vi "Micro-PL v10.4.0.vi"() -> ()   [LabVIEW 2010]
uses:
  drivers/Oxford ITC/ITCAPPS.LLB/ITCSetup.ctl
  drivers/Oxford ITC/ITCSUBS.LLB/ITCIO.ctl
  drivers/Oxford ITC/BUSGEN.LLB/OxfordAddress.ctl
  drivers/Oxford ITC/ITCSUBS.LLB/ITCVersion.ctl
  subvi/ESA-C/TypeDefs/ESA-C Live Controls.ctl
  subvi/ESA-C/TypeDefs/ESA-C Current Values.ctl
  subvi/ESA-C/TypeDefs/ESA-C Connection Settings.ctl
  subvi/ESA-C/TypeDefs/ESA-C Set Positions.ctl
  subvi/ITC503/TypeDefs/ITC503 Settings.ctl
  subvi/ITC503/TypeDefs/ITC503 Current Values.ctl
  subvi/iHR550/TypeDefs/iHR Current Values.ctl
  subvi/iHR550/TypeDefs/iHR Settings.ctl
  subvi/Mapping/TypeDefs/Mapping Spectra Params.ctl
  <vilib>/Utility/miscctls.llb/LVBoundsTypeDef.ctl
  <vilib>/Utility/miscctls.llb/LVPointTypeDef.ctl
  drivers/Horiba Spectrum One 3000V/Lib/CCD_command.llb/Comm Params.ctl
  subvi/Global Variables.vi
  <vilib>/Analysis/NI_AALBase.lvlib
panel:
  out "Spectrum Raw":dbl[][](array[numeric])
  out "Mapping State Storage":bool
  out "Mapping Reference":refnum<vi>
  out "Copy Drive Target":bool
  in  "CCD3500 Shutter":bool caption="Shutter:"
  out "ITC503 Temp Storage":dbl
  out "Runtime":u32
  out "ITC Gradient Time":i64
  out "Read ITC":bool
  out "Read CCD3500":bool
  out "Read iHR550":bool
  out "Read Drive":bool
  out "Spectrum Properties":cluster{"Position":T1, "Plot Area Size":T1}={"Position"={"Width"=36, "Height"=367}, "Plot Area Size"={"Width"=496, "Height"=264}}
  in  "Auto Folder":path caption="Ausgewählter Pfad"
  out "Int. Time Temp":dbl
  out "Wavelengths (nm)":dbl[](array[numeric])
  out "Measurement Running":bool
  out "ITC503s Running":bool
  out "Drive Running":bool
  out "CCD3500V Running":bool
  out "iHR550 Running":bool
  in  "Exit":bool
  out "iHR550 Status":bool
  out "Drive Status":bool
  out "CCD3500V Status":bool
  out "ITC503 Status":bool
  in  "CCD3500V Connection":T2={"Comm Interface"=1, "BUS"=0, "Address"=5, "Com Port"=0}
  out "Video Running":bool
  out "iHR550 RefNum":refnum<k7> caption="Mono RefNum out"
  out "ITC Setup":T3={"Description"="", "IO Info"={"Address"={"Com Port"=1, "ISOBUS Address"=1, "GPIB Address"=24, "Communication"=enum."ISOBUS"}, "Version"=enum."ITC503", "Ch 1 dec places"=1, "Ch 2 dec places"=1, "Ch 3 dec places"=1, "Ch1 Name"="", "Ch2 Name"="", "Ch3 Name"=""}}
  in  "Register":enum32{"Devices", "Acquisition / Mapping"}(tab)
  out "CCD3500 Temperature":dbl caption="Temp. (°C)" min=10.0 max=160.0 step=0.1 format="%.1f"
  in  "CCD3500V GPIB-Port":i32=5 caption="GPIB-Port" min=1 max=20 step=1 format="%#.0f"
  in  "CCD3500V Connect":bool
  out "CCD Timing":u32 caption="CCD"
  out "ITC Timing":u32 caption="ITC"
  out "Drive Timing":u32 caption="Drive"
  out "iHR550 Timing":u32 caption="iHR550"
  in  "iHR550 Force Init":bool=TRUE
  in  "iHR550 Connect":bool
  in  "iHR550 ID":string(combo)="iHR550" caption="Monochromator ID"
  out "ITC503 Current Values":T7 {"ITC503 Gradient" format="%.2f"; "ITC503 Setpoint" min=-273.0 max=300000.0 step=0.0001 format="%.1f"; "ITC503 I" format="%_1f"; "ITC503 P" format="%_1f"; "ITC503 Temperature" min=0.0 max=1645.0 step=1e-05 format="%.2f"; "ITC503 Heater" min=0.0 max=100.0 step=0.01 scale=0.0..100.0}
  in  "ITC503 Settings":T8={"ITC503 Set Setpoint"=0.0, "ITC503 Set Auto Heater"=TRUE, "ITC503 Set Auto PID"=TRUE, "P"=0.0, "I"=0.0, "D"=0.0} {"D" min=0.0 max=100.0 step=0.1 format="%.1f"; "I" min=0.0 max=100.0 step=0.1 format="%.1f"; "P" min=0.0 max=100.0 step=0.1 format="%.1f"; "ITC503 Set Setpoint" min=-273.0 max=300000.0 step=0.1 format="%.1f"}
  in  "ITC503 Configure":bool
  in  "ITC503 Connect":bool
  in  "ITC503 Selector":u16(ring) caption="Select Device" items=["ITC503s"]
  out "Drive Current Values":T9 {"Position"."Drive Z Position" min=-273.0 max=300000.0 step=0.0001 format="%.1f"; "Position"."Drive Y Position" min=-273.0 max=300000.0 step=0.0001 format="%.1f"; "Position"."Drive X Position" min=-273.0 max=300000.0 step=0.0001 format="%.1f"; "Voltages"."Drive Z Voltage" min=-273.0 max=300000.0 step=0.0001 format="%.1f"; "Voltages"."Drive Y Voltage" min=-273.0 max=300000.0 step=0.0001 format="%.1f"; "Voltages"."Drive X Voltage" min=-273.0 max=300000.0 step=0.0001 format="%.1f"}
  in  "Drive Connection":T10={"Objective GPIB-Port"=4, "Stage GPIB-Port"=4, "Drive Selector"=0, "Drive Velocity (V/s)"=5.0} {"Drive Velocity (V/s)" min=10.0 max=160.0 step=0.1 format="%.1f"; "Drive Selector" items=["Obj.", "Stage"]; "Stage GPIB-Port" min=1 max=20 step=1 format="%#.0f"; "Objective GPIB-Port" min=1 max=20 step=1 format="%#.0f"}
  in  "Drive Connect":bool
  in  "Spectrum Noise":i64 caption="Noise Level"
  in  "Wavelength Switch":bool
  out "Spectrum":cluster{dbl[], dbl[]}[](graph)
  in  "Spectrum Load":bool
  in  "Spectrum Save":bool
  in  "CCD3000 Current Rep.":string="0/0"
  in  "Spectrum Maximize":bool
  in  "Video Show":bool
  in  "Drive GoTo":bool caption="Objective Move Abs."
  in  "Drive New Positions":T11 {"Drive X Set" min=10.0 max=160.0 step=0.1 format="%.1f"; "Drive Z Set" min=10.0 max=160.0 step=0.1 format="%.1f"; "Drive Y Set" min=10.0 max=160.0 step=0.1 format="%.1f"}
  in  "Spectrum Autosave":bool caption="iHR550 Force Init"
  in  "CCD3500 Preview":bool
  in  "CCD3500 Acquire":bool
  in  "Spectra Settings":T12={"Integration Time"=1.0, "Repetitions"=1, "Mapping Spectra"=TRUE} caption="Mapping Spectra Settings" {"Repetitions" min=1 max=100 step=1; "Integration Time" min=0.1 max=6000.0 step=0.1 format="%.1f"}
  in  "Mapping Start":bool
  in  "iHR550 Configure":bool
  in  "iHR Settings":T13={"iHR550 Set Exit Mirror"=2, "iHR550 Set Side Exit"=0.0, "iHR550 Set Front Entrance"=0.0, "iHR550 Set Wavelength"=897.9988, "iHR550 Set Grating"=0, "iHR550 Set Grating Switch"=FALSE, "iHR550 Set Wavelength Switch"=FALSE, "iHR550 Set Mirror Switch"=FALSE, "iHR550 Set Slits Switch"=FALSE} {"iHR550 Set Grating" items=["1800"=1, "600"=2, "150"=3]; "iHR550 Set Wavelength" min=0.0 max=1500.0 step=1.0; "iHR550 Set Side Exit" min=0.0 max=2000.0 step=1.0; "iHR550 Set Exit Mirror" items=["Front"=2, "Side"=3]}
  out "iHR Current Values":T14={"iHR 550 Front Entrance"=0.0, "iHR550 Side Exit"=0.0, "iHR550 Wavelength"=897.9988, "iHR550 Exit Mirror"=2, "iHR550 Grating"="1", "Grating Index"=1} {"iHR550 Exit Mirror" items=["EntranceMirror", "ExitMirror", "Front", "Side"]}
  out "Drive Live Current Values":T9 {"Position"."Drive Z Position" min=-273.0 max=300000.0 step=0.0001 format="%.1f"; "Position"."Drive Y Position" min=-273.0 max=300000.0 step=0.0001 format="%.1f"; "Position"."Drive X Position" min=-273.0 max=300000.0 step=0.0001 format="%.1f"; "Voltages"."Drive Z Voltage" min=-273.0 max=300000.0 step=0.0001 format="%.1f"; "Voltages"."Drive Y Voltage" min=-273.0 max=300000.0 step=0.0001 format="%.1f"; "Voltages"."Drive X Voltage" min=-273.0 max=300000.0 step=0.0001 format="%.1f"}
  in  "Drive Live Controls":T15={"Snapshot"=FALSE, "Move Step"=1.0, "Move Home"=FALSE, "Move Down"=FALSE, "Move Up"=FALSE, "Move Left"=FALSE, "Move Right"=FALSE, "Move Out"=FALSE, "Move In"=FALSE} {"Move Step" min=0.0 max=30.0 step=0.1 format="%.1f"}
  # "Correlation Setup"
  # "Active"
  # "Active"
  # "ITC"
  # "iHR"
  # "Drive"
  # "CCD"
  # "Status"
  # "CCD"
  # "ITC"
  # "iHR"
  # "Drive"
  # "CCD"
  # "Timing"
  # "Monochromator"
  # "Cryostat"
  # "Drives"
  # "Drive Control"
  # "Spectrum"
  # "CCD"
  # "Mapping"
  # "Launch the Spectral Mapping VI and Raman Tool Set 2.0 in a new window."
  # "Monochromator"
  # "XY"
  # "Z"
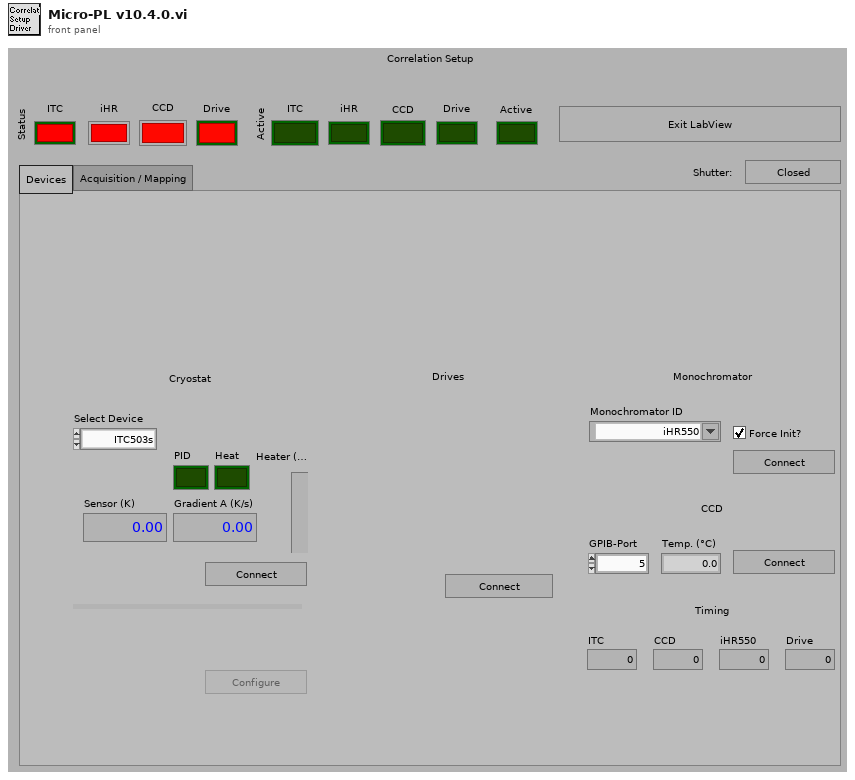
[diagram p1: front panel]
types:
  T1 = typedef "LVBoundsTypeDef.ctl" = cluster{"Width":u32, "Height":u32}
  T2 = cluster{"Comm Interface":u16, "BUS":i16, "Address":i16, "Com Port":i32}
  T3 = typedef "ITCSetup.ctl" = cluster{"Description":string, "IO Info":T4}
  T4 = typedef "ITCIO.ctl" = cluster{"Address":T5, "Version":T6, "Ch 1 dec places":i16, "Ch 2 dec places":i16, "Ch 3 dec places":i16, "Ch1 Name":string, "Ch2 Name":string, "Ch3 Name":string}
  T5 = typedef "OxfordAddress.ctl" = cluster{"Com Port":i32, "ISOBUS Address":i32, "GPIB Address":i16, "Communication":enum16{"RS232", "ISOBUS", "GPIB", "Gateway"}}
  T6 = typedef "ITCVersion.ctl" = enum16{"ITC502", "ITC503", "ITC601"}
  T7 = typedef "ITC503 Current Values.ctl" = cluster{"ITC503 Heater":dbl, "ITC503 Temperature":dbl, "ITC503 P":dbl, "ITC503 I":dbl, "ITC503 D":dbl, "ITC503 Setpoint":dbl, "ITC503 Gradient":dbl, "ITC503 Heater Auto":bool, "ITC503 PID Auto":bool}
  T8 = typedef "ITC503 Settings.ctl" = cluster{"ITC503 Set Setpoint":dbl, "ITC503 Set Auto Heater":bool, "ITC503 Set Auto PID":bool, "P":dbl, "I":dbl, "D":dbl}
  T9 = typedef "ESA-C Current Values.ctl" = cluster{"Voltages":cluster{"Drive X Voltage":dbl, "Drive Y Voltage":dbl, "Drive Z Voltage":dbl}, "Position":cluster{"Drive X Position":dbl, "Drive Y Position":dbl, "Drive Z Position":dbl}}
  T10 = typedef "ESA-C Connection Settings.ctl" = cluster{"Objective GPIB-Port":i32, "Stage GPIB-Port":i32, "Drive Selector":u16, "Drive Velocity (V/s)":dbl}
  T11 = typedef "ESA-C Set Positions.ctl" = cluster{"Drive X Set":dbl, "Drive Y Set":dbl, "Drive Z Set":dbl}
  T12 = typedef "Mapping Spectra Params.ctl" = cluster{"Integration Time":dbl, "Repetitions":u16, "Mapping Spectra":bool}
  T13 = typedef "iHR Settings.ctl" = cluster{"iHR550 Set Exit Mirror":u16, "iHR550 Set Side Exit":dbl, "iHR550 Set Front Entrance":dbl, "iHR550 Set Wavelength":dbl, "iHR550 Set Grating":u16, "iHR550 Set Grating Switch":bool, "iHR550 Set Wavelength Switch":bool, "iHR550 Set Mirror Switch":bool, "iHR550 Set Slits Switch":bool}
  T14 = typedef "iHR Current Values.ctl" = cluster{"iHR 550 Front Entrance":dbl, "iHR550 Side Exit":dbl, "iHR550 Wavelength":dbl, "iHR550 Exit Mirror":i32, "iHR550 Grating":string, "Grating Index":i32}
  T15 = typedef "ESA-C Live Controls.ctl" = cluster{"Snapshot":bool, "Move Step":dbl, "Move Home":bool, "Move Down":bool, "Move Up":bool, "Move Left":bool, "Move Right":bool, "Move Out":bool, "Move In":bool}
  T16 = typedef "LVPointTypeDef.ctl" = cluster{"Horizontal":i16, "Vertical":i16}
  T17 = enum8{"Enabled", "Disabled", "Disabled and Grayed Out"}
  T18 = typedef "Comm Params.ctl" = cluster{"Comm Interface":u16, "BUS":i16, "Address":i16, "Com Port":i32}
  T19 = enum16{"CCD Temperature Z345", "CCD Temperature Z308", "CCD Gain"}
  T20 = cluster{"CCD3000 Connection":T18, "Drive Connection Settings":T10, "ITC503 Current Values":T7, "Wavelengths (nm)":dbl[], "Drive Current Values":T9, "iHR Current Values":T14, "Spectra Settings":T12, "CCD3500 Temperature":dbl, "Simulate Drive 2":bool, "Simulate Spectra 2":bool}
  T21 = cluster{"Drive X Position":dbl, "Drive Y Position":dbl, "Drive Z Position":dbl}
  T22 = cluster{"Intensities":dbl[], "Wavelengths":dbl[]}[]
  T23 = typedef "LVPositionTypeDef.ctl" = cluster{"Left":i32, "Top":i32}
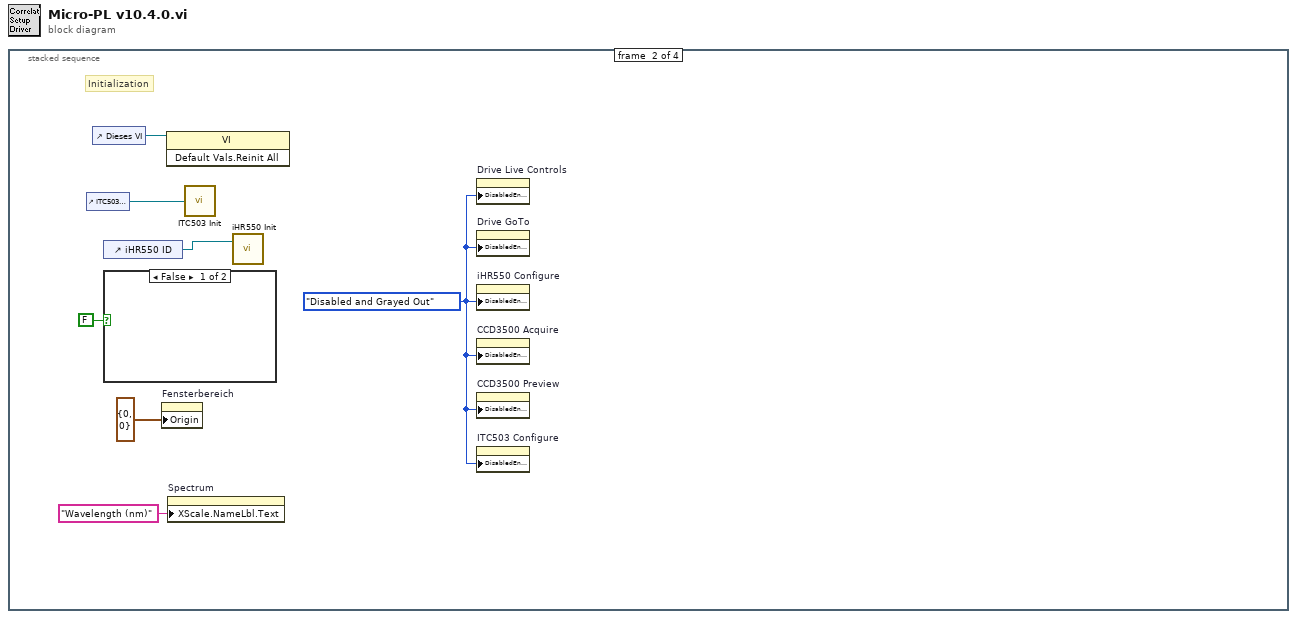
[diagram p0: block diagram]
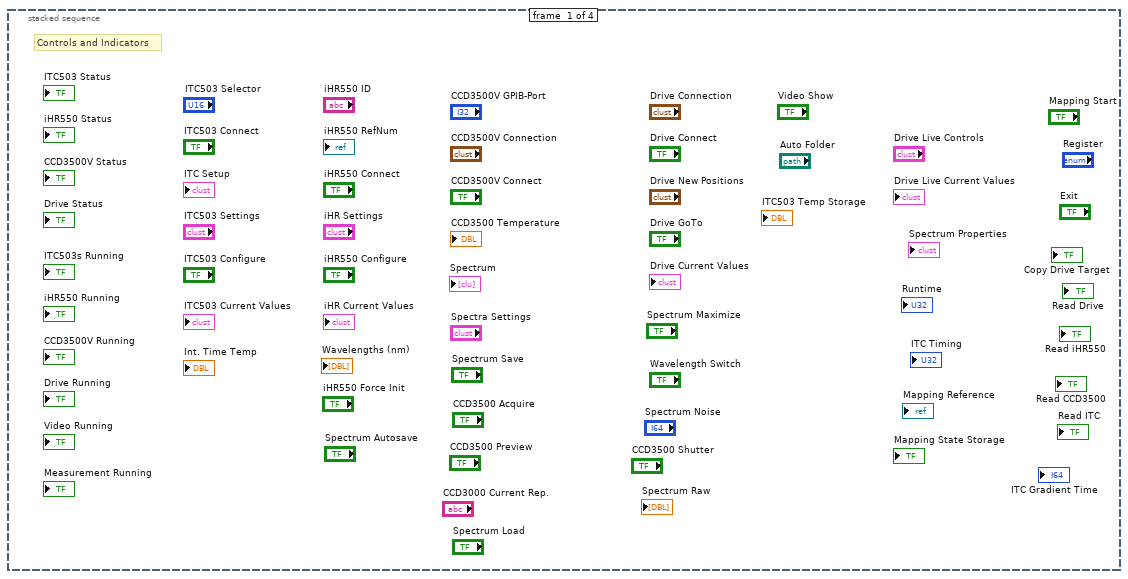
[diagram p2: hidden frame]
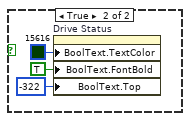
[diagram p3: hidden frame]
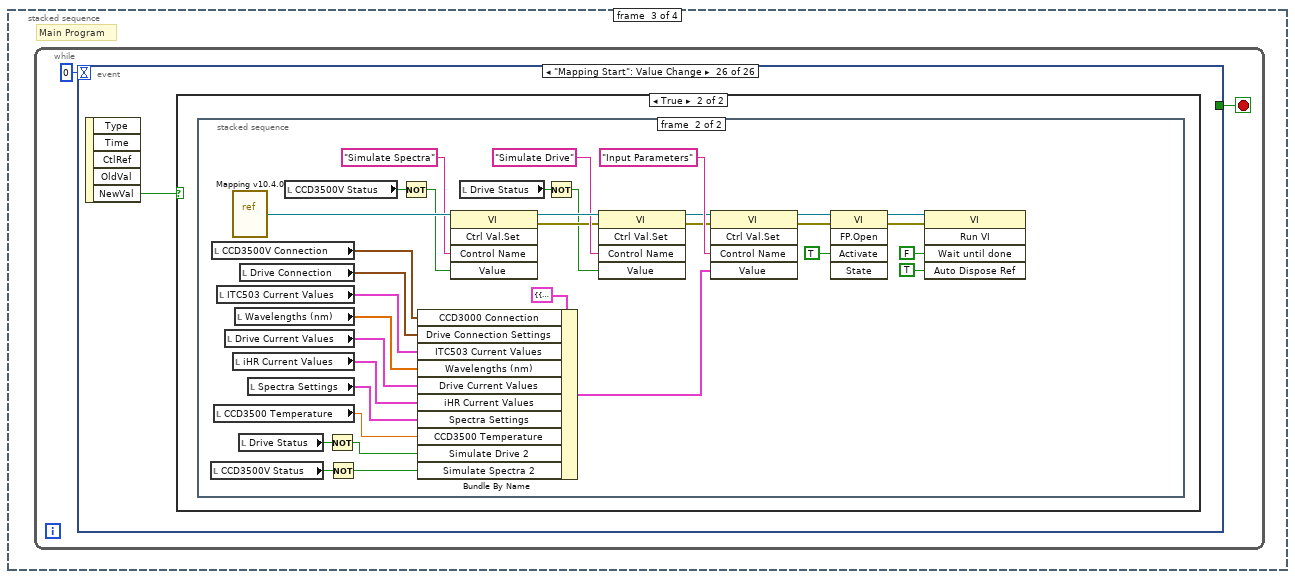
[diagram p4: hidden frame]
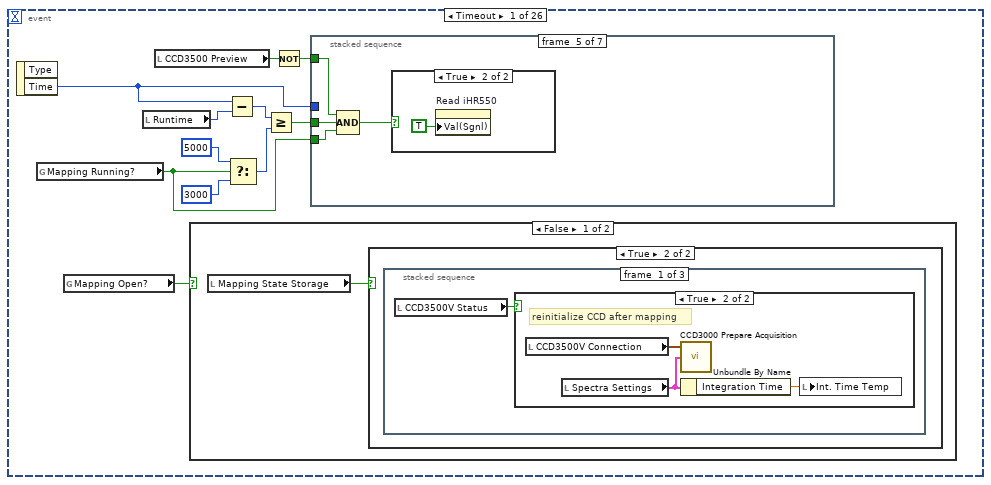
[diagram p5: hidden frame]
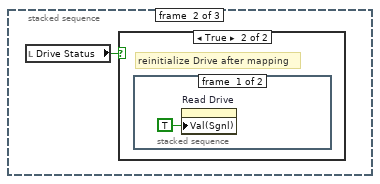
[diagram p8: hidden frame]
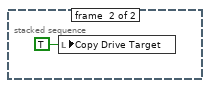
[diagram p10: hidden frame]
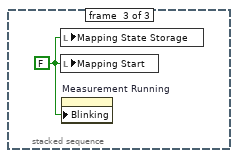
[diagram p11: hidden frame]
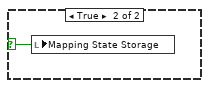
[diagram p12: hidden frame]
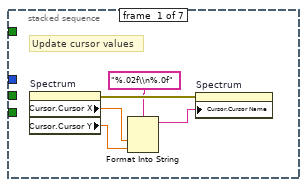
[diagram p13: hidden frame]
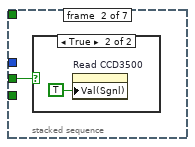
[diagram p14: hidden frame]
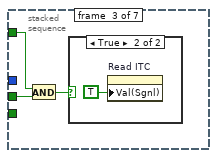
[diagram p16: hidden frame]
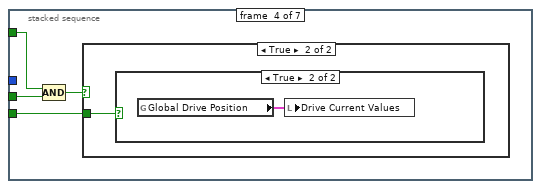
[diagram p18: hidden frame]
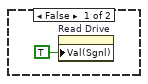
[diagram p20: hidden frame]
diagram:
  n1 = stacked-sequence {
    frame #0 {
      # "Controls and Indicators"
    }
    frame #1 {
      w2 = T17."Disabled and Grayed Out" ("Deaktiviert")
      # "Initialization"
      n2 = control-ref of="ITC503 Selector"() -> (w7:refnum<vi>)
      n3 = control-ref of="Dieses VI"() -> (w6:refnum<vi>)
      n4 = control-ref of="iHR550 ID"() -> (w5:refnum<vi>)
      n5 = case shown="False" FALSE {
        frame False {
        }
        frame True {
          n6 = property on="Drive Status" class="Bool (strict)"("BoolText.TextColor"=u32 15616, "BoolText.FontBold"=TRUE ("Boolescher Text.Schriftart:Fett"), "BoolText.Top"=-322 ("Boolescher Text.Position:Oben")) -> ()  [unwired: 2 in, 2 out]
        }
      }
      n7 = property on="Fensterbereich" class="Pane"("Origin"=T16 {"Horizontal"=0, "Vertical"=0}) -> ()  [unwired: 2 in, 2 out]
      n8 = invoke class="VI" method="Default Vals.Reinit All"(reference=w6) -> ()  [unwired: 2 in, 3 out]
      n9 = property on="Spectrum" class="XYGraph (strict)"("XScale.NameLbl.Text"="Wavelength (nm)" ("X Scale.Name Label.Text")) -> ()  [unwired: 2 in, 2 out]
      n10 = call "ITC503 Init.vi"("ITC Selector"=w7) -> ()  [unwired: 1 in]
      n11 = call "iHR550 Init.vi"("Mono ID"=w5) -> ()  [unwired: 2 in]
      n12 = property on="Drive Live Controls" class="Clust (strict)"("DisabledEnum"=w2) -> ()  [unwired: 2 in, 2 out]
      n13 = property on="Drive GoTo" class="Bool (strict)"("DisabledEnum"=w2) -> ()  [unwired: 2 in, 2 out]
      n14 = property on="iHR550 Configure" class="Bool (strict)"("DisabledEnum"=w2) -> ()  [unwired: 2 in, 2 out]
      n15 = property on="CCD3500 Acquire" class="Bool (strict)"("DisabledEnum"=w2) -> ()  [unwired: 2 in, 2 out]
      n16 = property on="CCD3500 Preview" class="Bool (strict)"("DisabledEnum"=w2) -> ()  [unwired: 2 in, 2 out]
      n17 = property on="ITC503 Configure" class="Bool (strict)"("DisabledEnum"=w2) -> ()  [unwired: 2 in, 2 out]
    }
    frame #2 {
      # "Main Program"
      n18 = while "Main-Program" {
        stop <- w12 stop-if-true
        n19 = event shown="[25] \"Mapping Start\": Value Change" {
          selector: _ -> [_ _ _ _ _ _ _ _ _ _ _ _ _ _ _ _ _ _ _ _ _ _ _ _ _ _]
          dyn-events: _ -> [_ _ _ _ _ _ _ _ _ _ _ _ _ _ _ _ _ _ _ _ _ _ _ _ _ _]
          timeout: 0 -> [_ _ _ _ _ _ _ _ _ _ _ _ _ _ _ _ _ _ _ _ _ _ _ _ _ _]
          tunnel: [_ w62 _ _ _ _ _ _ _ _ _ _ _ _ _ _ _ _ _ _ _ _ _ _ _ _] -> w12
          event Timeout {
            n20 = event-data() -> ("Time"=w19:u32)  [unwired: 1 in, 1 out]
            n21 = global read "Global Variables.vi" "Mapping Running?"() -> (w14:bool)
            n22 = global read "Global Variables.vi" "Mapping Open?"() -> (w13:bool)
            n23 = local read "Runtime"() -> (w18:u32)
            n24 = local read "CCD3500 Preview"() -> (w21:bool)
            n25 = case shown="False" w13 {
              selector: w13 -> [_ w33]
              frame False {
                n26 = local read "Mapping State Storage"() -> (w24:bool)
                n27 = case shown="True" w24 {
                  frame False {
                  }
                  frame True {
                    n28 = stacked-sequence {
                      frame #0 {
                        n29 = local read "CCD3500V Status"() -> (w25:bool)
                        n30 = case shown="True" w25 {
                          frame False {
                          }
                          frame True {
                            # "reinitialize CCD after mapping"
                            n31 = local read "CCD3500V Connection"() -> (w26:T2)
                            n32 = local read "Spectra Settings"() -> (w28:T12)
                            n33 = call "CCD3000 Prepare Acquisition.vi"("Mapping Spectra Settings"=w28, "Comm Params"=w26) -> ()  [unwired: 4 in]
                            n34 = Unbundle By Name(w28) -> ("Integration Time"=w27:dbl)
                            n35 = local write "Int. Time Temp"(w27) -> ()
                          }
                        }
                      }
                      frame #1 {
                        n36 = local read "Drive Status"() -> (w29:bool)
                        n37 = case shown="True" w29 {
                          frame False {
                          }
                          frame True {
                            # "reinitialize Drive after mapping"
                            n38 = stacked-sequence {
                              frame #0 {
                                n39 = property on="Read Drive" class="Bool (strict)"("Val(Sgnl)"=TRUE ("Value (Signaling)")) -> ()  [unwired: 2 in, 2 out]
                              }
                              frame #1 {
                                n40 = local write "Copy Drive Target"(TRUE ("Copy Drive Target")) -> ()
                              }
                            }
                          }
                        }
                      }
                      frame #2 {
                        w32 = FALSE ("Mapping Start")
                        n41 = local write "Mapping State Storage"(w32) -> ()
                        n42 = local write "Mapping Start"(w32) -> ()
                        n43 = property on="Measurement Running" class="Bool (strict)"("Blinking"=w32) -> ()  [unwired: 2 in, 2 out]
                      }
                    }
                  }
                }
              }
              frame True {
                n44 = local write "Mapping State Storage"(w33) -> ()
              }
            }
            n45 = Subtract(x=w19, y=w18) -> (x-y=w22:u32)
            n46 = Select(t=u32 5000 ("y"), s=w14, f=u32 3000 ("y")) -> (s? t:f=w15:u32)
            n47 = Greater Or Equal?(x=w22, y=w15) -> (x >= y?=w23:bool)
            n48 = Not(x=w21) -> (.not. x?=w20:bool)
            n49 = stacked-sequence {
              tunnel: w23 -> [_ w39 w43 w48 w55 _ w59]
              tunnel: w19 -> [_ _ _ _ _ _ w60]
              tunnel: w20 -> [_ _ w42 w47 w54 w57 _]
              tunnel: w14 -> [_ _ _ w45 w52 _ _]
              frame #0 {
                # "Update cursor values"
                n50 = property on="Spectrum" class="XYGraph (strict)"() -> (error out=w38:errorcluster, "Cursor.Cursor X"=w37:dbl, "Cursor.Cursor Y"=w36:dbl)  [unwired: 2 in, 1 out]
                n51 = Format Into String(format string="%.02f\\n%.0f", w37, w36) -> (resulting string=w34:string)  [unwired: 2 in, 1 out]
                n52 = property on="Spectrum" class="XYGraph (strict)"(error in=w38, "Cursor.Cursor Name"=w34) -> ()  [unwired: 1 in, 2 out]
              }
              frame #1 {
                n53 = case shown="True" w39 {
                  frame False {
                  }
                  frame True {
                    n54 = property on="Read CCD3500" class="Bool (strict)"("Val(Sgnl)"=TRUE ("Value (Signaling)")) -> ()  [unwired: 2 in, 2 out]
                  }
                }
              }
              frame #2 {
                n55 = And(x=w42, y=w43) -> (x .and. y?=w41:bool)
                n56 = case shown="True" w41 {
                  frame False {
                  }
                  frame True {
                    n57 = property on="Read ITC" class="Bool (strict)"("Val(Sgnl)"=TRUE ("Value (Signaling)")) -> ()  [unwired: 2 in, 2 out]
                  }
                }
              }
              frame #3 {
                n58 = Compound Arithmetic op=AND(w47, w48) -> (w46:bool)
                n59 = case shown="True" w46 {
                  tunnel: w45 -> [_ w49]
                  frame False {
                  }
                  frame True {
                    n60 = case shown="True" w49 {
                      frame False {
                        n61 = property on="Read Drive" class="Bool (strict)"("Val(Sgnl)"=TRUE ("Value (Signaling)")) -> ()  [unwired: 2 in, 2 out]
                      }
                      frame True {
                        n62 = global read "Global Variables.vi" "Global Drive Position"() -> (w51:T9)
                        n63 = local write "Drive Current Values"(w51) -> ()
                      }
                    }
                  }
                }
              }
              frame #4 {
                n64 = Compound Arithmetic op=AND(w54, w55, w52) -> (w53:bool)
                n65 = case shown="True" w53 {
                  frame False {
                  }
                  frame True {
                    n66 = property on="Read iHR550" class="Bool (strict)"("Val(Sgnl)"=TRUE ("Value (Signaling)")) -> ()  [unwired: 2 in, 2 out]
                  }
                }
              }
              frame #5 {
                n67 = case shown="False" w57 {
                  frame False {
                    n68 = property on="CCD3500 Acquire" class="Bool (strict)"("Val(Sgnl)"=TRUE ("Wert (signalisierend)")) -> ()  [unwired: 2 in, 2 out]
                  }
                  frame True {
                  }
                }
              }
              frame #6 {
                # "Set runtime counter"
                n69 = case shown="True" w59 {
                  tunnel: w60 -> [_ w61]
                  frame False {
                  }
                  frame True {
                    n70 = local write "Runtime"(w61) -> ()
                  }
                }
              }
            }
          }
          event "Exit": Value Change {
            n71 = event-data() -> ("NewVal"=w62:bool)  [unwired: 1 in, 4 out]
          }
          event "ITC503 Connect": Value Change {
            n72 = event-data() -> ("NewVal"=w63:bool)  [unwired: 1 in, 4 out]
            n73 = stacked-sequence {
              tunnel: w63 -> [_ w65 _]
              frame #0 {
                n74 = property on="ITC503s Running" class="Bool (strict)"("Blinking"=TRUE ("Blinkend")) -> ()  [unwired: 2 in, 2 out]
              }
              frame #1 {
                n75 = case shown="True" w65 {
                  selector: w65 -> [w70 _]
                  tunnel: [w70 w77] -> w67
                  frame False {
                    # "disconnect"
                    n76 = control-ref of="ITC503s Running"() -> (w71:refnum<vi>)
                    n77 = property class="Bool (strict)"(reference=w71, "Blinking"=w70, "Value"=w70) -> ()  [unwired: 1 in, 2 out]
                  }
                  frame True {
                    # "connect"
                    n78 = local read "ITC503 Selector"() -> (w78:u16)
                    n79 = call "ITC503 Connect.vi"("ITC Selector"=w78) -> ("ITC Setup"=w76:T3, "Connected"=w77:bool)
                    n80 = local write "ITC Setup"(w76) -> ()
                    n81 = call "ITC503 Get Values.vi"("ITC Setup"=w76) -> ("ITC503 Current Values"=w75:T7)  [unwired: 1 in, 1 out]
                    n82 = Unbundle By Name(w75) -> ("ITC503 Setpoint"=w72:dbl)
                    n83 = Bundle By Name(cluster=T8 {"ITC503 Set Setpoint"=0.0, "ITC503 Set Auto Heater"=TRUE, "ITC503 Set Auto PID"=TRUE, "P"=0.0, "I"=0.0, "D"=0.0} ("ITC503 Settings"), "ITC503 Set Setpoint"=w72) -> (w73:T8)
                    n84 = local write "ITC503 Settings"(w73) -> ()
                  }
                }
                n85 = case shown="False" w67 {
                  tunnel: [T17."Disabled and Grayed Out" ("Deaktiviert") T17."Enabled" ("Deaktiviert")] -> w66
                  frame False {
                  }
                  frame True {
                  }
                }
                n86 = local write "ITC503 Status"(w67) -> ()
                n87 = local write "ITC503 Connect"(w67) -> ()
                n88 = property on="ITC503 Configure" class="Bool (strict)"("DisabledEnum"=w66) -> ()  [unwired: 2 in, 2 out]
              }
              frame #2 {
                n89 = property on="ITC503s Running" class="Bool (strict)"("Blinking"=FALSE ("Blinkend")) -> ()  [unwired: 2 in, 2 out]
                n90 = property on="Read ITC" class="Bool (strict)"("Val(Sgnl)"=TRUE ("Wert (signalisierend)")) -> ()  [unwired: 2 in, 2 out]
              }
            }
          }
          event "Read ITC": Value Change {
            n91 = event-data() -> ("Time"=w82:u32, "NewVal"=w86:bool)  [unwired: 1 in, 3 out]
            n92 = local read "ITC503 Status"() -> (w85:bool)
            n93 = control-ref of="ITC503s Running"() -> (w83:refnum<vi>)
            n94 = And(x=w85, y=w86) -> (x .and. y?=w84:bool)
            n95 = case shown="True" w84 {
              tunnel: w83 -> [w88 w92]
              tunnel: w82 -> [_ w91]
              tunnel: [u32 0 w90] -> w81
              frame False {
                n96 = property class="Bool (strict)"(reference=w88, "BoolText.Text"="" ("Boolescher Text.Text")) -> ()  [unwired: 1 in, 2 out]
              }
              frame True {
                n97 = stacked-sequence {
                  seq-local: [_ w98 _ _] -> [_ _ w114 _]
                  seq-local: [w93 _ _ _] -> [_ _ _ w120]
                  tunnel: w92 -> [_ _ w107 _]
                  tunnel: w91 -> [_ w99 _ _]
                  tunnel: [_ _ _ w121] -> w90
                  frame #0 {
                    n98 = Tick Count (ms)() -> (millisecond timer value=w93:u32)
                  }
                  frame #1 {
                    n99 = local read "ITC Setup"() -> (w105:T3)
                    n100 = local read "ITC Gradient Time"() -> (w103:i64)
                    n101 = call "ITC503 Get Values.vi"("ITC Setup"=w105) -> ("ITC503 Current Values"=w98:T7)  [unwired: 1 in, 1 out]
                    n102 = local read "ITC503 Temp Storage"() -> (w97:dbl)
                    n103 = Unbundle By Name(w98) -> ("ITC503 Temperature"=w95:dbl)
                    n104 = Subtract(x=w99, y=w103) -> (x-y=w102:i64)
                    n105 = Divide(x=w102, y=i64 1000) -> (x/y=w100:dbl)
                    n106 = Subtract(x=w95, y=w97) -> (x-y=w96:dbl)
                    n107 = Divide(x=w96, y=w100) -> (x/y=w104:dbl)
                    n108 = Bundle By Name(cluster=w98, "ITC503 Gradient"=w104) -> (w94:T7)
                    n109 = local write "ITC503 Current Values"(w94) -> ()
                    n110 = global write "Global Variables.vi" "Global ITC Values"(w94) -> ()
                  }
                  frame #2 {
                    n111 = Unbundle By Name(w114) -> ("ITC503 Temperature"=w106:dbl, "ITC503 Setpoint"=w115:dbl)
                    n112 = Subtract(x=w106, y=w115) -> (x-y=w116:dbl)
                    n113 = Number To Fractional String(number=w106, precision (6)=i16 2 ("Genauigkeit (6)")) -> (F-format string=w110:string)  [unwired: 2 in]
                    n114 = Absolute Value(x=w116) -> (abs(x)=w117:dbl)
                    n115 = String Subset(string=w110, length (rest)=5 ("Länge (Rest)")) -> (substring=w108:string)  [unwired: 1 in]
                    n116 = Greater?(x=w117, y=2.0) -> (0:w113:bool)
                    n117 = Not(x=w113) -> (.not. x?=w112:bool)
                    n118 = property class="Bool (strict)"(reference=w107, "Blinking"=w113, "Value"=w112, "BoolText.Text"=w108) -> ()  [unwired: 1 in, 2 out]
                    n119 = local write "ITC503 Temp Storage"(w106) -> ()
                  }
                  frame #3 {
                    n120 = Tick Count (ms)() -> (millisecond timer value=w119:u32)
                    n121 = local write "ITC Gradient Time"(w119) -> ()
                    n122 = Subtract(x=w119, y=w120) -> (x-y=w121:u32)
                  }
                }
              }
            }
            n123 = local write "ITC Timing"(w81) -> ()
          }
          event "iHR550 Connect": Value Change {
            n124 = event-data() -> ("NewVal"=w122:bool)  [unwired: 1 in, 4 out]
            n125 = stacked-sequence {
              tunnel: w122 -> [_ w125 _]
              frame #0 {
                n126 = property on="iHR550 Running" class="Bool (strict)"("Blinking"=TRUE ("Blinkend")) -> ()  [unwired: 2 in, 2 out]
              }
              frame #1 {
                n127 = case shown="True" w125 {
                  selector: w125 -> [w129 _]
                  tunnel: [w129 w142] -> w124
                  frame False {
                    # "disconnect"
                  }
                  frame True {
                    # "connect"
                    n128 = local read "iHR550 Force Init"() -> (w140:bool)
                    n129 = control-ref of="iHR550 Set Grating"() -> (w141:refnum<vi>)
                    n130 = local read "iHR550 ID"() -> (w143:string)
                    n131 = call "iHR550 Connect.vi"("Force\nInitialization"=w140, "Grating Selector"=w141, "Mono ID"=w143) -> ("Initialized"=w142:bool, "iHR550 RefNum"=w139:refnum<k7>)  [unwired: 2 in, 4 out]
                    n132 = local write "iHR550 RefNum"(w139) -> ()
                    n133 = call "iHR550 Read Values.vi"("JYMONOLib.IJYMonoReqd"=w139) -> ("iHR Current Values"=w131:T14)  [unwired: 1 in]
                    n134 = local write "iHR Current Values"(w131) -> ()
                    n135 = Unbundle By Name(w131) -> ("iHR 550 Front Entrance"=w137:dbl, "iHR550 Side Exit"=w136:dbl, "iHR550 Wavelength"=w135:dbl, "iHR550 Exit Mirror"=w134:i32, "Grating Index"=w132:i32)
                    n136 = call "iHR550 Convert Axis.vi"("iHR Current Values"=w131) -> ("Wavelengths (nm)"=w130:dbl[])
                    n137 = local write "Wavelengths (nm)"(w130) -> ()
                    n138 = Bundle By Name(cluster=T13 {"iHR550 Set Exit Mirror"=0, "iHR550 Set Side Exit"=0.0, "iHR550 Set Front Entrance"=0.0, "iHR550 Set Wavelength"=0.0, "iHR550 Set Grating"=0, "iHR550 Set Grating Switch"=FALSE, "iHR550 Set Wavelength Switch"=FALSE, "iHR550 Set Mirror Switch"=FALSE, "iHR550 Set Slits Switch"=FALSE} ("iHR Settings"), "iHR550 Set Front Entrance"=w137, "iHR550 Set Side Exit"=w136, "iHR550 Set Wavelength"=w135, "iHR550 Set Exit Mirror"=w134, "iHR550 Set Grating"=w132) -> (w133:T13)
                    n139 = local write "iHR Settings"(w133) -> ()
                  }
                }
                n140 = local write "iHR550 Status"(w124) -> ()
                n141 = local write "iHR550 Connect"(w124) -> ()
                n142 = case shown="False" w124 {
                  tunnel: [T17."Disabled and Grayed Out" ("Deaktiviert") T17."Enabled" ("Deaktiviert")] -> w126
                  frame False {
                  }
                  frame True {
                  }
                }
                n143 = property on="iHR550 Configure" class="Bool (strict)"("DisabledEnum"=w126) -> ()  [unwired: 2 in, 2 out]
              }
              frame #2 {
                n144 = local write "iHR550 Force Init"(FALSE ("iHR550 Force Init")) -> ()
                n145 = property on="iHR550 Running" class="Bool (strict)"("Blinking"=FALSE ("Blinkend")) -> ()  [unwired: 2 in, 2 out]
                n146 = property on="Read iHR550" class="Bool (strict)"("Val(Sgnl)"=TRUE ("Wert (signalisierend)")) -> ()  [unwired: 2 in, 2 out]
              }
            }
          }
          event "Read iHR550": Value Change {
            n147 = event-data() -> ("NewVal"=w150:bool)  [unwired: 1 in, 4 out]
            n148 = local read "iHR550 Status"() -> (w149:bool)
            n149 = And(x=w149, y=w150) -> (x .and. y?=w148:bool)
            n150 = case shown="True" w148 {
              tunnel: [u32 0 w152] -> w147
              frame False {
              }
              frame True {
                n151 = stacked-sequence {
                  seq-local: [w153 _ _] -> [_ _ w156]
                  tunnel: [_ _ w157] -> w152
                  frame #0 {
                    n152 = Tick Count (ms)() -> (millisecond timer value=w153:u32)
                  }
                  frame #1 {
                    n153 = local read "iHR550 RefNum"() -> (w155:refnum<k7>)
                    n154 = call "iHR550 Read Values.vi"("JYMONOLib.IJYMonoReqd"=w155) -> ("iHR Current Values"=w154:T14)  [unwired: 1 in]
                    n155 = local write "iHR Current Values"(w154) -> ()
                    n156 = global write "Global Variables.vi" "Global iHR Values"(w154) -> ()
                  }
                  frame #2 {
                    n157 = Tick Count (ms)() -> (millisecond timer value=w158:u32)
                    n158 = Subtract(x=w158, y=w156) -> (x-y=w157:u32)
                  }
                }
              }
            }
            "iHR550 Timing" <- w147
          }
          event "CCD3500V Connect": Value Change {
            n159 = event-data() -> ("NewVal"=w159:bool)  [unwired: 1 in, 4 out]
            n160 = stacked-sequence {
              tunnel: w159 -> [_ w161 _]
              frame #0 {
                n161 = property on="CCD3500V Running" class="Bool (strict)"("Blinking"=TRUE ("Blinkend")) -> ()  [unwired: 2 in, 2 out]
              }
              frame #1 {
                n162 = case shown="True" w161 {
                  selector: w161 -> [w167 _]
                  tunnel: [w167 w168] -> w163
                  frame False {
                    # "disconnect"
                    n163 = local read "CCD3500V Connection"() -> (w166:T2)
                    n164 = call "CCDSTOP.VI"("Comm Params"=w166) -> ()  [unwired: 1 out]
                  }
                  frame True {
                    # "connect"
                    n165 = stacked-sequence {
                      seq-local: [_ w172 _] -> [_ _ w174]
                      tunnel: [_ w173 _] -> w168
                      frame #0 {
                        n166 = local read "CCD3500V GPIB-Port"() -> (w170:i32)
                        n167 = Bundle By Name(cluster=T18 {"Comm Interface"=1, "BUS"=0, "Address"=5, "Com Port"=1} ("Comm Params"), "Address"=w170) -> (w171:T18)
                        n168 = local write "CCD3500V Connection"(w171) -> ()
                      }
                      frame #1 {
                        n169 = local read "CCD3500V Connection"() -> (w172:T2)
                        n170 = call "CCD3000 Initialize.vi"("Comm Params"=w172) -> ("Success"=w173:bool)  [unwired: 9 in, 1 out]
                      }
                      frame #2 {
                        n171 = local read "Spectra Settings"() -> (w175:T12)
                        n172 = Unbundle By Name(w175) -> ("Integration Time"=w176:dbl)
                        n173 = local write "Int. Time Temp"(w176) -> ()
                        n174 = call "CCD3000 Prepare Acquisition.vi"("Mapping Spectra Settings"=w175, "Comm Params"=w174) -> ()  [unwired: 4 in]
                      }
                    }
                  }
                }
                n175 = local write "CCD3500V Connect"(w163) -> ()
                n176 = local write "CCD3500V Status"(w163) -> ()
                n177 = case shown="False" w163 {
                  tunnel: [T17."Disabled and Grayed Out" ("Deaktiviert") T17."Enabled" ("Deaktiviert")] -> w162
                  frame False {
                  }
                  frame True {
                  }
                }
                n178 = property on="CCD3500V Status" class="Bool (strict)"("BoolText.Visible"=w163) -> ()  [unwired: 2 in, 2 out]
                n179 = property on="CCD3500 Acquire" class="Bool (strict)"("DisabledEnum"=w162) -> ()  [unwired: 2 in, 2 out]
                n180 = property on="CCD3500 Preview" class="Bool (strict)"("DisabledEnum"=w162) -> ()  [unwired: 2 in, 2 out]
              }
              frame #2 {
                n181 = property on="Read CCD3500" class="Bool (strict)"("Val(Sgnl)"=TRUE ("Wert (signalisierend)")) -> ()  [unwired: 2 in, 2 out]
                n182 = property on="CCD3500V Running" class="Bool (strict)"("Blinking"=FALSE ("Blinkend")) -> ()  [unwired: 2 in, 2 out]
              }
            }
          }
          event "Read CCD3500": Value Change {
            n183 = event-data() -> ("NewVal"=w182:bool)  [unwired: 1 in, 4 out]
            n184 = local read "CCD3500V Status"() -> (w181:bool)
            n185 = And(x=w181, y=w182) -> (x .and. y?=w180:bool)
            n186 = case shown="True" w180 {
              tunnel: [u32 0 w184] -> w179
              frame False {
              }
              frame True {
                n187 = stacked-sequence {
                  seq-local: [_ w186 _ _] -> [_ _ w191 _]
                  seq-local: [w185 _ _ _] -> [_ _ _ w202]
                  tunnel: [_ _ _ w203] -> w184
                  frame #0 {
                    n188 = Tick Count (ms)() -> (millisecond timer value=w185:u32)
                  }
                  frame #1 {
                    n189 = local read "CCD3500V Connection"() -> (w190:T2)
                    n190 = call "PROPGET.VI"("CCD Prop ID"=T19."CCD Temperature Z345", "Comm Params"=w190) -> ("Output Param"=w188:dbl)  [unwired: 1 out]
                    n191 = Subtract(x=w188, y=273.15) -> (x-y=w186:dbl)
                    n192 = local write "CCD3500 Temperature"(w186) -> ()
                  }
                  frame #2 {
                    n193 = Greater?(x=w191, y=-122.0) -> (0:w192:bool)
                    n194 = case shown="True" w192 {
                      selector: w192 -> [w199 w201]
                      tunnel: [cluster{u32, u32}[] [{16713728, 16713728}, {6618880, 6618880}] ("Farben [4]") cluster{u32, u32}[] [{16713728, 16713728}] ("Farben [4]")] -> w193
                      tunnel: [w199 w201] -> w195
                      frame False {
                      }
                      frame True {
                      }
                    }
                    n195 = Number To Fractional String(number=w191, precision (6)=i16 1 ("Genauigkeit (6)")) -> (F-format string=w194:string)  [unwired: 2 in]
                    n196 = global write "Global Variables.vi" "Global CCD Temperature (C)"(w191) -> ()
                    n197 = property on="CCD3500V Status" class="Bool (strict)"("Blinking"=w195, "BoolText.Text"=w194, "Colors [4]"=w193) -> ()  [unwired: 2 in, 2 out]
                  }
                  frame #3 {
                    n198 = Tick Count (ms)() -> (millisecond timer value=w204:u32)
                    n199 = Subtract(x=w204, y=w202) -> (x-y=w203:u32)
                  }
                }
              }
            }
            "CCD Timing" <- w179
          }
          event "Drive Connect": Value Change {
            n200 = event-data() -> ("NewVal"=w205:bool)  [unwired: 1 in, 4 out]
            n201 = stacked-sequence {
              tunnel: w205 -> [_ w209 _ _]
              frame #0 {
                n202 = property on="Drive Running" class="Bool (strict)"("Blinking"=TRUE ("Blinkend")) -> ()  [unwired: 2 in, 2 out]
              }
              frame #1 {
                n203 = local read "Drive Connection"() -> (w210:T10)
                n204 = Not(x=w209) -> (.not. x?=w211:bool)
                n205 = call "ESA-C Connect.vi"("Remote=F /Local=T"=w211, "Drive Connection Settings"=w210) -> ("Success"=w212:bool)  [unwired: 2 in]
                n206 = Exclusive Or(1:w211, 2:w212) -> (0:w213:bool)
                n207 = local write "Drive Connect"(w213) -> ()
                n208 = local write "Drive Status"(w213) -> ()
                n209 = case shown="False" w213 {
                  tunnel: [T17."Disabled and Grayed Out" ("Deaktiviert") T17."Enabled" ("Deaktiviert")] -> w208
                  tunnel: ["" ("Boolescher Text.Text") w216] -> w207
                  frame False {
                  }
                  frame True {
                    n210 = property on="Drive Selector" class="Ring (strict)"() -> ("RingText.Text"=w216:string)  [unwired: 2 in, 2 out]
                  }
                }
                n211 = property on="Drive Live Controls" class="Clust (strict)"("DisabledEnum"=w208) -> ()  [unwired: 2 in, 2 out]
                n212 = property on="Drive Status" class="Bool (strict)"("BoolText.Text"=w207) -> ()  [unwired: 2 in, 2 out]
                n213 = property on="Drive GoTo" class="Bool (strict)"("DisabledEnum"=w208) -> ()  [unwired: 2 in, 2 out]
              }
              frame #2 {
                # "prepare mirroring values to target controls"
                n214 = local write "Copy Drive Target"(TRUE ("Copy Drive Target")) -> ()
              }
              frame #3 {
                n215 = property on="Drive Running" class="Bool (strict)"("Blinking"=FALSE ("Blinkend")) -> ()  [unwired: 2 in, 2 out]
                n216 = property on="Read Drive" class="Bool (strict)"("Val(Sgnl)"=TRUE ("Wert (signalisierend)")) -> ()  [unwired: 2 in, 2 out]
              }
            }
          }
          event "Read Drive": Value Change {
            n217 = event-data() -> ("NewVal"=w224:bool)  [unwired: 1 in, 4 out]
            n218 = local read "Drive Status"() -> (w223:bool)
            n219 = And(x=w223, y=w224) -> (x .and. y?=w222:bool)
            n220 = case shown="True" w222 {
              tunnel: [u32 0 w226] -> w221
              frame False {
              }
              frame True {
                n221 = stacked-sequence {
                  seq-local: [w227 _ _ _] -> [_ _ _ w233]
                  tunnel: [_ _ _ w232] -> w226
                  frame #0 {
                    n222 = Tick Count (ms)() -> (millisecond timer value=w227:u32)
                  }
                  frame #1 {
                    n223 = local read "Drive Connection"() -> (w229:T10)
                    n224 = call "ESA-C Get Values.vi"("Drive Connection Settings"=w229) -> ("Drive Current Values"=w228:T9)
                    n225 = local write "Drive Live Current Values"(w228) -> ()
                    n226 = local write "Drive Current Values"(w228) -> ()
                    n227 = global write "Global Variables.vi" "Global Drive Position"(w228) -> ()
                  }
                  frame #2 {
                    n228 = local read "Copy Drive Target"() -> (w230:bool)
                    n229 = case shown="True" w230 {
                      frame False {
                      }
                      frame True {
                        n230 = property on="Copy Drive Target" class="Bool (strict)"("Val(Sgnl)"=TRUE ("Value (Signaling)")) -> ()  [unwired: 2 in, 2 out]
                      }
                    }
                  }
                  frame #3 {
                    n231 = Tick Count (ms)() -> (millisecond timer value=w234:u32)
                    n232 = Subtract(x=w234, y=w233) -> (x-y=w232:u32)
                  }
                }
              }
            }
            "Drive Timing" <- w221
          }
          event "Copy Drive Target": Value Change {
            # "this event is triggered after drive readout\nit should usually not be triggered directly by signaling"
            n233 = event-data() -> ("NewVal"=w235:bool)  [unwired: 1 in, 4 out]
            n234 = case shown="True" w235 {
              frame False {
              }
              frame True {
                n235 = stacked-sequence {
                  frame #0 {
                    n236 = local read "Drive Current Values"() -> (w237:T9)
                    n237 = Unbundle By Name(w237) -> ("Position"=w236:T21)
                    n238 = local write "Drive New Positions"(w236) -> ()
                  }
                  frame #1 {
                    n239 = local write "Copy Drive Target"(FALSE ("Copy Drive Target")) -> ()
                  }
                }
              }
            }
          }
          event "Video Show": Value Change {
            n240 = event-data() -> ("NewVal"=w239:bool)  [unwired: 1 in, 4 out]
            n241 = case shown="False" w239 {
              frame False {
                n242 = call "Video Close.vi"() -> ()  [unwired: 11 in, 1 out]
              }
              frame True {
                n243 = call "Video Open.vi"() -> ()  [unwired: 11 in, 1 out]
              }
            }
          }
          event "ITC503 Configure": Value Change {
            n244 = event-data() -> ("NewVal"=w240:bool)  [unwired: 1 in, 4 out]
            n245 = stacked-sequence {
              tunnel: w240 -> [_ w242 _]
              frame #0 {
                n246 = property on="ITC503s Running" class="Bool (strict)"("Blinking"=TRUE ("Blinkend")) -> ()  [unwired: 2 in, 2 out]
              }
              frame #1 {
                n247 = local read "ITC503 Status"() -> (w244:bool)
                n248 = And(x=w244, y=w242) -> (x .and. y?=w243:bool)
                n249 = case shown="True" w243 {
                  frame False {
                  }
                  frame True {
                    n250 = local read "ITC503 Settings"() -> (w245:T8)
                    n251 = local read "ITC Setup"() -> (w246:T3)
                    n252 = call "ITC503 Set Values.vi"("Set Channel"=i16 1, "ITC503 Settings"=w245, "ITC Setup"=w246) -> ()  [unwired: 2 in]
                  }
                }
              }
              frame #2 {
                w249 = FALSE ("Blinkend")
                n253 = local write "ITC503 Configure"(w249) -> ()
                n254 = property on="ITC503s Running" class="Bool (strict)"("Blinking"=w249) -> ()  [unwired: 2 in, 2 out]
                n255 = property on="Read ITC" class="Bool (strict)"("Val(Sgnl)"=TRUE ("Wert (signalisierend)")) -> ()  [unwired: 2 in, 2 out]
              }
            }
          }
          event "iHR550 Configure": Value Change {
            n256 = event-data() -> ("NewVal"=w250:bool)  [unwired: 1 in, 4 out]
            n257 = stacked-sequence {
              tunnel: w250 -> [_ w252 _]
              frame #0 {
                n258 = property on="iHR550 Running" class="Bool (strict)"("Blinking"=TRUE ("Blinkend")) -> ()  [unwired: 2 in, 2 out]
              }
              frame #1 {
                n259 = local read "iHR550 Status"() -> (w254:bool)
                n260 = local read "iHR550 RefNum"() -> (w255:refnum<k7>)
                n261 = And(x=w254, y=w252) -> (x .and. y?=w253:bool)
                n262 = case shown="True" w253 {
                  tunnel: w255 -> [_ w256]
                  frame False {
                  }
                  frame True {
                    n263 = stacked-sequence {
                      seq-local: [_ w261 _] -> [_ _ w264]
                      tunnel: w256 -> [w257 w262 _]
                      frame #0 {
                        w260 = u16 2 items=["Front"=2, "Side"=3] ("Entrance Mirror")
                        n264 = local read "iHR Settings"() -> (w258:T13)
                        n265 = call "iHR550 Set Values.vi"("Refnum out"=w257, "Entrance Mirror"=w260, "Target\nSide Entrance"=0.0 ("Target\nSide Entrance"), "iHR Settings"=w258) -> ()  [unwired: 11 in, 1 out]
                      }
                      frame #1 {
                        n266 = call "iHR550 Read Values.vi"("JYMONOLib.IJYMonoReqd"=w262) -> ("iHR Current Values"=w261:T14)  [unwired: 1 in]
                        n267 = local write "iHR Current Values"(w261) -> ()
                      }
                      frame #2 {
                        n268 = call "iHR550 Convert Axis.vi"("iHR Current Values"=w264) -> ("Wavelengths (nm)"=w263:dbl[])
                        n269 = local write "Wavelengths (nm)"(w263) -> ()
                        n270 = global write "Global Variables.vi" "Global Wavelengths (nm)"(w263) -> ()
                      }
                    }
                  }
                }
              }
              frame #2 {
                w266 = FALSE ("Blinkend")
                n271 = property on="Read iHR550" class="Bool (strict)"("Val(Sgnl)"=TRUE ("Wert (signalisierend)")) -> ()  [unwired: 2 in, 2 out]
                n272 = local write "iHR550 Configure"(w266) -> ()
                n273 = property on="iHR550 Running" class="Bool (strict)"("Blinking"=w266) -> ()  [unwired: 2 in, 2 out]
              }
            }
          }
          event "CCD3500 Preview": Value Change {
            n274 = event-data() -> ("NewVal"=w267:bool)  [unwired: 1 in, 4 out]
            n275 = case shown="True" w267 {
              frame False {
              }
              frame True {
                n276 = property on="CCD3500 Acquire" class="Bool (strict)"("Val(Sgnl)"=TRUE ("Wert (signalisierend)")) -> ()  [unwired: 2 in, 2 out]
              }
            }
          }
          event "CCD3500 Acquire": Value Change {
            n277 = event-data() -> ("NewVal"=w269:bool)  [unwired: 1 in, 4 out]
            n278 = stacked-sequence {
              tunnel: w269 -> [w270 _]
              frame #0 {
                n279 = case shown="True" w270 {
                  frame False {
                  }
                  frame True {
                    n280 = local read "CCD3500V Connection"() -> (w271:T2)
                    n281 = local read "Spectra Settings"() -> (w272:T12)
                    n282 = stacked-sequence {
                      tunnel: w272 -> [w275 w287 _]
                      tunnel: w271 -> [w274 w283 _]
                      frame #0 {
                        # "prepare acquisition if settings changed"
                        n283 = Unbundle By Name(w275) -> ("Integration Time"=w273:dbl)
                        n284 = local read "Int. Time Temp"() -> (w276:dbl)
                        n285 = Equal?(x=w273, y=w276) -> (x = y?=w277:bool)
                        n286 = case shown="False" w277 {
                          tunnel: w276 -> [_ _]
                          tunnel: w275 -> [w280 _]
                          tunnel: w274 -> [w279 _]
                          tunnel: w273 -> [w278 _]
                          frame False {
                            n287 = call "CCD3000 Prepare Acquisition.vi"("Mapping Spectra Settings"=w280, "Comm Params"=w279) -> ()  [unwired: 4 in]
                            n288 = local write "Int. Time Temp"(w278) -> ()
                          }
                          frame True {
                          }
                        }
                      }
                      frame #1 {
                        n289 = local read "CCD3500 Preview"() -> (w286:bool)
                        n290 = Unbundle By Name(w287) -> ("Repetitions"=w284:u16)
                        n291 = Select(t=i8 1, s=w286, f=w284) -> (s? t:f=w282:u16)
                        n292 = for {
                          N: w282 -> [w297]
                          tunnel: w283 -> [w309]
                          shift-right: [w304] -> _
                          shift-left: u16[][] [] -> [w307]
                          i -> [w298]
                          stop <- w303 continue-if-true
                          n293 = control-ref of="CCD3500 Acquire"() -> (w302:refnum<vi>)
                          n294 = control-ref of="CCD3500V Running"() -> (w301:refnum<vi>)
                          n295 = call "CCD3000 Spectral Acquisition.vi"("Acquire"=w302, "Running"=w301, "Comm Params"=w309) -> ("Raw-Spectrum"=w308:u16[])  [unwired: 6 in, 2 out]
                          n296 = Number To Decimal String(number=w297) -> (decimal integer string=w296:string)  [unwired: 1 in]
                          n297 = Build Array (concatenate)(w308, w307) -> (w304:u16[][])
                          n298 = Increment(x=w298) -> (x+1=w294:i32)
                          n299 = Number To Decimal String(number=w294) -> (decimal integer string=w295:string)  [unwired: 1 in]
                          n300 = local read "Wavelengths (nm)"() -> (w306:dbl[])
                          n301 = local read "Spectrum Noise"() -> (w293:i64)
                          n302 = Concatenate Strings(w295, "/" ("string"), w296) -> (w300:string)
                          n303 = call "CCD3000 Average Spectra.vi"("Repetitions"=w294, "Raw Spectra"=w304) -> ("Raw Spectrum"=w305:dbl[])
                          n304 = local read "Wavelength Switch"() -> (w292:bool)
                          n305 = local write "CCD3000 Current Rep."(w300) -> ()
                          n306 = call "CCD3000 Pixel to Wavelength v10.1.0.vi"("Wavelengths (nm)"=w306, "Raw Spectrum"=w305) -> ("Spectrum-Array"=w288:dbl[][])  [unwired: 1 out]
                          n307 = call "CCD3000 Noise Subtraction v10.4.0.vi"("Spectrum Noise"=w293, "Spectrum-Array In"=w288) -> ("Spectrum-Array Out"=w291:dbl[][], "Spectrum-Cluster"=w289:T22)
                          n308 = local write "Spectrum Raw"(w288) -> ()
                          n309 = case shown="False" w292 {
                            tunnel: w291 -> [_ w312]
                            tunnel: [w310 w311] -> w290
                            tunnel: w289 -> [w310 _]
                            frame False {
                            }
                            frame True {
                              n310 = call "CCD3000 Jacobian Transformation v10.4.0.vi"("Spectrum-Array In"=w312) -> ("Spectrum-Cluster"=w311:T22)  [unwired: 1 in, 1 out]
                            }
                          }
                          n311 = local read "CCD3500 Acquire"() -> (w303:bool)
                          n312 = local write "Spectrum"(w290) -> ()
                        }
                      }
                      frame #2 {
                        n313 = local read "Spectrum Autosave"() -> (w313:bool)
                        n314 = case shown="True" w313 {
                          frame False {
                          }
                          frame True {
                            n315 = property on="Spectrum Save" class="Bool (strict)"("Val(Sgnl)"=TRUE ("Value (Signaling)")) -> ()  [unwired: 2 in, 2 out]
                          }
                        }
                      }
                    }
                  }
                }
              }
              frame #1 {
                n316 = local write "CCD3500 Acquire"(FALSE ("Blinkend")) -> ()
                n317 = local write "CCD3000 Current Rep."("0/0" ("CCD3000 Current Rep.")) -> ()
              }
            }
          }
          event "Wavelength Switch": Value Change {
            n318 = event-data() -> ("NewVal"=w317:bool)  [unwired: 1 in, 4 out]
            n319 = case shown="False" w317 {
              frame False {
                n320 = local read "Spectrum Noise"() -> (w318:i64)
                n321 = local read "Spectrum Raw"() -> (w319:dbl[][])
                n322 = property on="Spectrum" class="XYGraph (strict)"("XScale.NameLbl.Text"="Wavelenght (nm)" ("X Scale.Name Label.Text")) -> ()  [unwired: 2 in, 2 out]
                n323 = call "CCD3000 Noise Subtraction v10.4.0.vi"("Spectrum Noise"=w318, "Spectrum-Array In"=w319) -> ("Spectrum-Cluster"=w320:T22)  [unwired: 1 out]
                n324 = local write "Spectrum"(w320) -> ()
              }
              frame True {
                # "Jacobian Transformation requires noise subtraction"
                n325 = local read "Spectrum Noise"() -> (w323:i64)
                n326 = Greater Than 0?(x=w323) -> (x > 0?=w322:bool)
                n327 = case shown="True" w322 {
                  frame False {
                    n328 = local write "Wavelength Switch"(FALSE ("Wavelength Switch")) -> ()
                    n329 = call "Display Message to User"() -> ()  [unwired: 10 in, 2 out]
                  }
                  frame True {
                    n330 = local read "Spectrum Noise"() -> (w325:i64)
                    n331 = local read "Spectrum Raw"() -> (w326:dbl[][])
                    n332 = property on="Spectrum" class="XYGraph (strict)"("XScale.NameLbl.Text"="Energy (eV)" ("X Scale.Name Label.Text")) -> ()  [unwired: 2 in, 2 out]
                    n333 = call "CCD3000 Noise Subtraction v10.4.0.vi"("Spectrum Noise"=w325, "Spectrum-Array In"=w326) -> ("Spectrum-Array Out"=w327:dbl[][])  [unwired: 1 out]
                    n334 = call "CCD3000 Jacobian Transformation v10.4.0.vi"("Spectrum-Array In"=w327) -> ("Spectrum-Cluster"=w328:T22)  [unwired: 1 in, 1 out]
                    n335 = local write "Spectrum"(w328) -> ()
                  }
                }
              }
            }
          }
          event "Spectrum Noise": Value Change {
            n336 = event-data() -> ("NewVal"=w331:i64)  [unwired: 1 in, 4 out]
            n337 = Greater Than 0?(x=w331) -> (x > 0?=w330:bool)
            n338 = stacked-sequence {
              tunnel: w330 -> [w332 _]
              frame #0 {
                n339 = case shown="True" w332 {
                  frame False {
                    # "Disable Jacobian Transformation"
                    n340 = local write "Wavelength Switch"(FALSE ("Wavelength Switch")) -> ()
                  }
                  frame True {
                  }
                }
              }
              frame #1 {
                n341 = local read "Wavelength Switch"() -> (w334:bool)
                n342 = local read "Spectrum Noise"() -> (w339:i64)
                n343 = local read "Spectrum Raw"() -> (w338:dbl[][])
                n344 = call "CCD3000 Noise Subtraction v10.4.0.vi"("Spectrum Noise"=w339, "Spectrum-Array In"=w338) -> ("Spectrum-Array Out"=w337:dbl[][], "Spectrum-Cluster"=w335:T22)
                n345 = case shown="False" w334 {
                  tunnel: w337 -> [_ w342]
                  tunnel: [w340 w341] -> w336
                  tunnel: w335 -> [w340 _]
                  frame False {
                  }
                  frame True {
                    n346 = call "CCD3000 Jacobian Transformation v10.4.0.vi"("Spectrum-Array In"=w342) -> ("Spectrum-Cluster"=w341:T22)  [unwired: 1 in, 1 out]
                  }
                }
                n347 = local write "Spectrum"(w336) -> ()
              }
            }
          }
          event "CCD3500 Shutter": Value Change {
            n348 = event-data() -> ("NewVal"=w343:bool)  [unwired: 1 in, 4 out]
            n349 = local read "CCD3500V Status"() -> (w344:bool)
            n350 = case shown="True" w344 {
              tunnel: w343 -> [_ w347]
              frame False {
              }
              frame True {
                n351 = local read "CCD3500V Connection"() -> (w346:T2)
                n352 = call "CCD Shutter.vi"("Shutter"=w347, "Comm Params"=w346) -> ("Error"=w345:bool)
                n353 = case shown="True" w345 {
                  tunnel: w347 -> [_ w348]
                  frame False {
                  }
                  frame True {
                    n354 = Not(x=w348) -> (.not. x?=w349:bool)
                    n355 = local write "CCD3500 Shutter"(w349) -> ()
                  }
                }
              }
            }
          }
          event "Drive GoTo": Value Change {
            n356 = event-data() -> ("NewVal"=w350:bool)  [unwired: 1 in, 4 out]
            n357 = stacked-sequence {
              tunnel: w350 -> [_ w352 _]
              frame #0 {
                n358 = property on="Drive Running" class="Bool (strict)"("Blinking"=TRUE ("Blinkend")) -> ()  [unwired: 2 in, 2 out]
              }
              frame #1 {
                n359 = local read "Drive Status"() -> (w354:bool)
                n360 = And(x=w354, y=w352) -> (x .and. y?=w353:bool)
                n361 = case shown="True" w353 {
                  frame False {
                  }
                  frame True {
                    n362 = local read "Drive New Positions"() -> (w355:T11)
                    n363 = local read "Drive Connection"() -> (w356:T10)
                    n364 = control-ref of="Drive Running"() -> (w357:refnum<vi>)
                    n365 = call "ESA-C Move Absolute.vi"("Running"=w357, "Drive New Abs. Positions"=w355, "Drive Connection Settings"=w356) -> ()  [unwired: 2 in]
                  }
                }
              }
              frame #2 {
                w359 = FALSE ("Blinkend")
                n366 = local write "Drive GoTo"(w359) -> ()
                n367 = property on="Drive Running" class="Bool (strict)"("Blinking"=w359) -> ()  [unwired: 2 in, 2 out]
                n368 = property on="Read Drive" class="Bool (strict)"("Val(Sgnl)"=TRUE ("Wert (signalisierend)")) -> ()  [unwired: 2 in, 2 out]
              }
            }
          }
          event Value Change {
            n369 = event-data() -> ("NewVal"=w361:bool)  [unwired: 1 in, 4 out]
            n370 = local read "Drive Status"() -> (w362:bool)
            n371 = And(x=w362, y=w361) -> (x .and. y?=w360:bool)
            n372 = case shown="True" w360 {
              frame False {
              }
              frame True {
                n373 = stacked-sequence {
                  seq-local: [w363 _ _ _] -> [_ w379 _ _]
                  frame #0 {
                    # "Move and Read"
                    n374 = flat-sequence {
                      tunnel: [w370] -> w366
                      tunnel: [w367] -> w365
                      tunnel: w366 -> [w372]
                      tunnel: w365 -> [w373]
                      tunnel: [w371] -> w364
                      tunnel: w364 -> [w378]
                      tunnel: [w378] -> w363
                      frame #0 {
                        n375 = local read "Drive Live Controls"() -> (w367:T15)
                        n376 = local read "Drive Connection"() -> (w368:T10)
                        n377 = control-ref of="Drive Running"() -> (w369:refnum<vi>)
                        n378 = call "ESA-C Live Control.vi"("Running"=w369, "Drive Live Controls"=w367, "Drive Connection Settings"=w368) -> ("Reset Switches"=w370:bool)  [unwired: 1 in]
                      }
                      frame #1 {
                        n379 = case shown="True" w372 {
                          tunnel: w373 -> [w374 w377]
                          tunnel: [w374 w376] -> w371
                          frame False {
                          }
                          frame True {
                            w375 = FALSE ("Move Out")
                            n380 = Bundle By Name(cluster=w377, "Move Home"=w375, "Move Down"=w375, "Move Up"=w375, "Move Left"=w375, "Move Right"=w375, "Move Out"=w375, "Move In"=w375) -> (w376:T15)
                          }
                        }
                      }
                      frame #2 {
                        n381 = local write "Drive Live Controls"(w378) -> ()
                      }
                    }
                  }
                  frame #1 {
                    # "Snapshot"
                    n382 = Unbundle By Name(w379) -> ("Snapshot"=w382:bool)
                    n383 = case shown="True" w382 {
                      selector: w382 -> [w383 _]
                      tunnel: [w383 FALSE] -> w381
                      frame False {
                      }
                      frame True {
                        n384 = call "Video Snapshot.vi"() -> ()  [unwired: 11 in, 1 out]
                      }
                    }
                    n385 = Bundle By Name(cluster=w379, "Snapshot"=w381) -> (w380:T15)
                    n386 = local write "Drive Live Controls"(w380) -> ()
                  }
                  frame #2 {
                    n387 = local write "Copy Drive Target"(TRUE ("Copy Drive Target")) -> ()
                  }
                  frame #3 {
                    n388 = property on="Read Drive" class="Bool (strict)"("Val(Sgnl)"=TRUE ("Wert (signalisierend)")) -> ()  [unwired: 2 in, 2 out]
                  }
                }
              }
            }
          }
          event "Spectrum Save": Value Change {
            n389 = event-data() -> ("NewVal"=w387:bool)  [unwired: 1 in, 4 out]
            n390 = stacked-sequence {
              tunnel: w387 -> [w388 _]
              frame #0 {
                n391 = case shown="True" w388 {
                  frame False {
                  }
                  frame True {
                    n392 = local read "CCD3500 Temperature"() -> (w394:dbl)
                    n393 = local read "ITC503 Current Values"() -> (w395:T7)
                    n394 = local read "Drive Current Values"() -> (w396:T9)
                    n395 = local read "iHR Current Values"() -> (w398:T14)
                    n396 = local read "Spectra Settings"() -> (w397:T12)
                    n397 = local read "Spectrum Raw"() -> (w389:dbl[][])
                    n398 = call "Export_spectrumFileName.vi"("ITC503 Current Values"=w395, "iHR Current Values"=w398, "Spectra Settings"=w397, "Drive Current Values"=w396, "CCD3500 Temperature"=w394) -> ("Filename"=w393:string)
                    n399 = local read "Spectrum Autosave"() -> (w391:bool)
                    n400 = local read "Auto Folder"() -> (w390:path)
                    n401 = call "Export_2DtoTxt v10.2.0.vi"("Auto Folder"=w390, "Auto?"=w391, "Data (2D)"=w389, "Export Type"="Spectrum", "Filename"=w393) -> ()  [unwired: 1 in]
                  }
                }
              }
              frame #1 {
                n402 = local write "Spectrum Save"(FALSE ("Spectrum Save")) -> ()
              }
            }
          }
          event "Spectrum Load": Value Change {
            n403 = event-data() -> ("NewVal"=w400:bool)  [unwired: 1 in, 4 out]
            n404 = case shown="True" w400 {
              frame False {
              }
              frame True {
                n405 = stacked-sequence {
                  seq-local: [w401 _ _] -> [_ w404 _]
                  frame #0 {
                    n406 = call "Load Spectrum.vi"() -> ("Intensity"=w401:dbl[], "Wavelength"=w403:dbl[])  [unwired: 3 in, 1 out]
                    n407 = Build Array(w403, w401) -> (w402:dbl[][])
                    n408 = local write "Spectrum Raw"(w402) -> ()
                  }
                  frame #1 {
                    n409 = call <vilib>:"Median.vi"("X"=w404) -> ("median"=w406:dbl)  [unwired: 1 out]
                    n410 = To Long Integer(number=w406) -> (32bit integer=w405:i32)
                    n411 = property on="Spectrum Noise" class="DigNum (strict)"("Val(Sgnl)"=w405) -> ()  [unwired: 2 in, 2 out]
                  }
                  frame #2 {
                    n412 = local write "Spectrum Load"(FALSE ("Spectrum Load")) -> ()
                  }
                }
              }
            }
          }
          event "Spectrum Autosave": Value Change {
            n413 = event-data() -> ("NewVal"=w409:bool)  [unwired: 1 in, 4 out]
            n414 = case shown="True" w409 {
              tunnel: [path "" w415] -> w408
              frame False {
              }
              frame True {
                n415 = call "File Dialog"("prompt"="Choose Save Folder") -> ("selected path"=w417:path, "cancelled"=w411:bool, "error out"=w413:errorcluster)  [unwired: 11 in, 1 out]
                n416 = call <vilib>:"Simple Error Handler.vi"("error in (no error)"=w413) -> ("error?"=w412:bool)  [unwired: 4 in, 4 out]
                n417 = Or(x=w411, y=w412) -> (x .or. y?=w414:bool)
                n418 = case shown="True" w414 {
                  tunnel: w417 -> [w418 _]
                  tunnel: [w418 path ""] -> w415
                  frame False {
                  }
                  frame True {
                    n419 = local write "Spectrum Autosave"(FALSE ("Spectrum Autosave")) -> ()
                  }
                }
              }
            }
            n420 = local write "Auto Folder"(w408) -> ()
          }
          event "Spectrum Maximize": Value Change {
            n421 = event-data() -> ("NewVal"=w421:bool)  [unwired: 1 in, 4 out]
            n422 = case shown="True" w421 {
              frame False {
                n423 = local read "Spectrum Properties"() -> (w424:cluster{"Position":T1, "Plot Area Size":T1})
                n424 = Unbundle(w424) -> ("Position"=w423:T1, "Plot Area Size"=w422:T1)
                n425 = stacked-sequence {
                  tunnel: w423 -> [_ w426]
                  tunnel: w422 -> [w425 _]
                  frame #0 {
                    n426 = property on="Spectrum" class="XYGraph (strict)"("Plot Area Size"=w425) -> ()  [unwired: 2 in, 2 out]
                  }
                  frame #1 {
                    n427 = property on="Spectrum" class="XYGraph (strict)"("Position"=w426) -> ()  [unwired: 2 in, 2 out]
                  }
                }
              }
              frame True {
                n428 = property on="Spectrum" class="XYGraph (strict)"() -> ("Bounds"=w447:T1, "Plot Area Size"=w446:T1, "Position"=w444:T23)  [unwired: 2 in, 2 out]
                n429 = Bundle("Position"=w444, "Plot Area Size"=w446) -> (w445:cluster{"Position":T23, "Plot Area Size":T1})  [unwired: 1 in]
                n430 = Unbundle By Name(w447) -> ("Width"=w451:u32, "Height"=w452:u32)
                n431 = Unbundle By Name(w446) -> ("Width"=w454:u32, "Height"=w453:u32)
                n432 = property on="Register" class="TabCtl (strict)"() -> ("Bounds"=w450:T1, "Position"=w439:T23, "Width"=w430:u32, "Height"=w429:u32)  [unwired: 2 in, 2 out]
                n433 = local write "Spectrum Properties"(w445) -> ()
                n434 = Subtract(x=w451, y=w454) -> (x-y=w443:u32)
                n435 = Subtract(x=w452, y=w453) -> (x-y=w440:u32)
                n436 = Add(x=w443, y=u32 25) -> (x+y=w442:u32)
                n437 = Add(x=w440, y=u32 70) -> (x+y=w441:u32)
                n438 = Subtract(x=w430, y=w442) -> (x-y=w449:u32)
                n439 = Subtract(x=w429, y=w441) -> (x-y=w448:u32)
                n440 = Bundle By Name(cluster=w450, "Width"=w449, "Height"=w448) -> (w427:T1)
                n441 = Unbundle By Name(w439) -> ("Left"=w438:i32, "Top"=w435:i32)
                n442 = Add(x=w438, y=20) -> (x+y=w437:i32)
                n443 = Add(x=w435, y=50) -> (x+y=w436:i32)
                n444 = Bundle By Name(cluster=w439, "Left"=w437, "Top"=w436) -> (w428:T23)
                n445 = stacked-sequence {
                  tunnel: w428 -> [w455 _]
                  tunnel: w427 -> [_ w456]
                  frame #0 {
                    n446 = property on="Spectrum" class="XYGraph (strict)"("Position"=w455) -> ()  [unwired: 2 in, 2 out]
                  }
                  frame #1 {
                    n447 = property on="Spectrum" class="XYGraph (strict)"("Plot Area Size"=w456) -> ()  [unwired: 2 in, 2 out]
                  }
                }
              }
            }
          }
          event "Mapping Start": Value Change {
            n448 = event-data() -> ("NewVal"=w457:bool)  [unwired: 1 in, 4 out]
            n449 = case shown="True" w457 {
              frame False {
              }
              frame True {
                n450 = stacked-sequence {
                  frame #0 {
                    n451 = property on="Measurement Running" class="Bool (strict)"("Blinking"=TRUE ("Blinkend")) -> ()  [unwired: 2 in, 2 out]
                  }
                  frame #1 {
                    n452 = local read "CCD3500V Status"() -> (w480:bool)
                    n453 = local read "CCD3500V Connection"() -> (w489:T2)
                    n454 = local read "CCD3500 Temperature"() -> (w491:dbl)
                    n455 = local read "ITC503 Current Values"() -> (w486:T7)
                    n456 = local read "Drive Current Values"() -> (w484:T9)
                    n457 = vi-ref "Mapping v10.4.0.vi"() -> (w469:refnum<vi>)
                    n458 = local read "iHR Current Values"() -> (w485:T14)
                    n459 = local read "Wavelengths (nm)"() -> (w487:dbl[])
                    n460 = local read "Drive Status"() -> (w482:bool)
                    n461 = local read "Drive Connection"() -> (w488:T10)
                    n462 = local read "Spectra Settings"() -> (w490:T12)
                    n463 = local read "CCD3500V Status"() -> (w462:bool)
                    n464 = Not(x=w482) -> (.not. x?=w481:bool)
                    n465 = Not(x=w480) -> (.not. x?=w479:bool)
                    n466 = Not(x=w462) -> (.not. x?=w461:bool)
                    n467 = Bundle By Name(cluster=T20 {"CCD3000 Connection"={"Comm Interface"=1, "BUS"=0, "Address"=5, "Com Port"=1}, "Drive Connection Settings"={"Objective GPIB-Port"=4, "Stage GPIB-Port"=4, "Drive Selector"=0, "Drive Velocity (V/s)"=5.0}, "ITC503 Current Values"={"ITC503 Heater"=0.0, "ITC503 Temperature"=0.0, "ITC503 P"=0.0, "ITC503 I"=0.0, "ITC503 D"=0.0, "ITC503 Setpoint"=0.0, "ITC503 Gradient"=0.0, "ITC503 Heater Auto"=FALSE, "ITC503 PID Auto"=FALSE}, "Wavelengths (nm)"=[], "Drive Current Values"={"Voltages"={"Drive X Voltage"=0.0, "Drive Y Voltage"=0.0, "Drive Z Voltage"=0.0}, "Position"={"Drive X Position"=0.0, "Drive Y Position"=0.0, "Drive Z Position"=0.0}}, "iHR Current Values"={"iHR 550 Front Entrance"=0.0, "iHR550 Side Exit"=0.0, "iHR550 Wavelength"=897.9988, "iHR550 Exit Mirror"=2, "iHR550 Grating"="1", "Grating Index"=1}, "Spectra Settings"={"Integration Time"=1.0, "Repetitions"=1, "Mapping Spectra"=TRUE}, "CCD3500 Temperature"=0.0, "Simulate Drive 2"=FALSE, "Simulate Spectra 2"=FALSE} ("Input Parameters"), "CCD3000 Connection"=w489, "Drive Connection Settings"=w488, "ITC503 Current Values"=w486, "Wavelengths (nm)"=w487, "Drive Current Values"=w484, "iHR Current Values"=w485, "Spectra Settings"=w490, "CCD3500 Temperature"=w491, "Simulate Drive 2"=w481, "Simulate Spectra 2"=w479) -> (w470:T20)
                    n468 = invoke class="VI" method="Ctrl Val.Set"(reference=w469, "Control Name"="Simulate Spectra", "Value"=w461) -> (reference out=w468:refnum<vi>, error out=w463:errorcluster)  [unwired: 2 in, 3 out]
                    n469 = local read "Drive Status"() -> (w460:bool)
                    n470 = Not(x=w460) -> (.not. x?=w459:bool)
                    n471 = invoke class="VI" method="Ctrl Val.Set"(reference=w468, error in=w463, "Control Name"="Simulate Drive", "Value"=w459) -> (reference out=w467:refnum<vi>, error out=w464:errorcluster)  [unwired: 1 in, 3 out]
                    n472 = invoke class="VI" method="Ctrl Val.Set"(reference=w467, error in=w464, "Control Name"="Input Parameters", "Value"=w470) -> (reference out=w471:refnum<vi>, error out=w472:errorcluster)  [unwired: 1 in, 3 out]
                    n473 = invoke on="Invoke Node" class="VI" method="FP.Open"(reference=w471, error in=w472, "Activate"=TRUE ("Activate?")) -> (reference out=w474:refnum<vi>, error out=w473:errorcluster)  [unwired: 2 in, 3 out]
                    n474 = invoke on="Invoke Node" class="VI" method="Run VI"(reference=w474, error in=w473, "Wait until done"=FALSE ("Wait Until Done"), "Auto Dispose Ref"=TRUE ("Auto Dispose Reference")) -> ()  [unwired: 1 in, 5 out]
                  }
                }
              }
            }
          }
        }
      }
    }
    frame #3 {
      # "Close Connections"
      n475 = control-ref of="Dieses VI"() -> (w492:refnum<vi>)
      n476 = invoke class="VI" method="Default Vals.Reinit All"(reference=w492) -> ()  [unwired: 2 in, 3 out]
    }
  }
